vi "Sample Rate Trigger.vi"(8 "SampleDelay(in)":u32, 9 "Sample Rate (Hz)":dbl, 11 "Last Event mS":u32) -> (0 "Boolean":bool, 3 "Last Event mS":u32, 4 "Elapsed mS":u32, 6 "SampleDelay":u32)   [LabVIEW 2021]
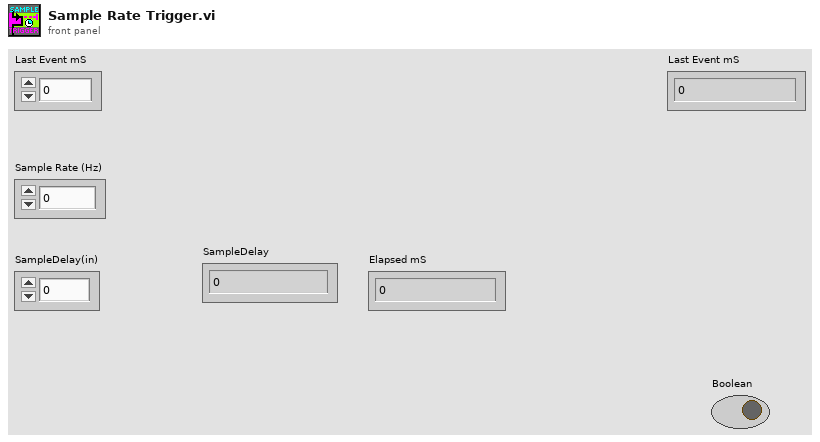
[diagram p1: front panel]
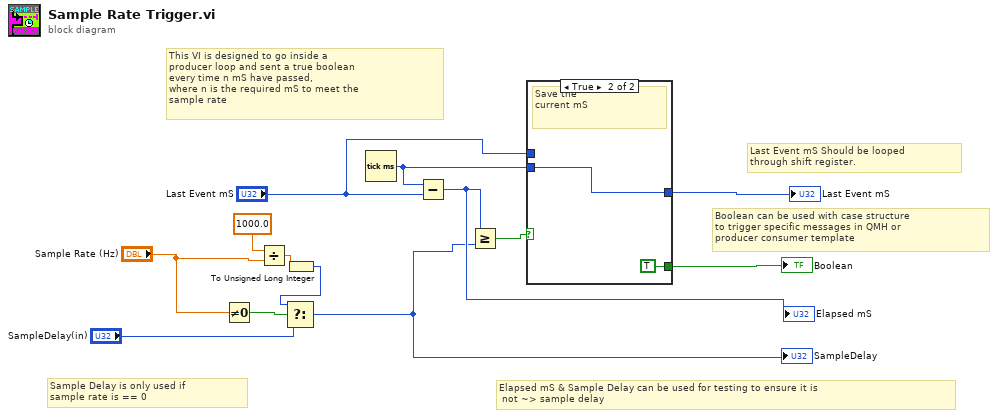
[diagram p0: block diagram]
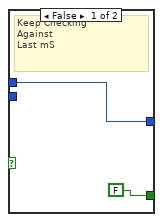
[diagram p2: hidden frame]
diagram:
  # "Sample Delay is only used if\nsample rate is == 0"
  # "Elapsed mS & Sample Delay can be used for testing to ensure it is\n not ~> sample delay"
  # "Boolean can be used with case structure\nto trigger specific messages in QMH or \nproducer consumer template"
  # "This VI is designed to go inside a\nproducer loop and sent a true boolean\nevery time n mS have passed, \nwhere n is the required mS to meet the \nsample rate"
  # "Last Event mS Should be looped\nthrough shift register."
  n1 = Not Equal To 0?(x="Sample Rate (Hz)") -> (x != 0?=w4:bool)
  n2 = Divide(x=1000.0, y="Sample Rate (Hz)") -> (x/y=w8:dbl)
  n3 = To Unsigned Long Integer(number=w8) -> (unsigned 32bit integer=w2:u32)
  n4 = Select(t=w2, s=w4, f="SampleDelay(in)") -> (s? t:f=w3:u32)
  "SampleDelay" <- w3
  n5 = Tick Count (ms)() -> (millisecond timer value=w11:u32)
  n6 = Subtract(x=w11, y="Last Event mS") -> (x-y=w6:u32)
  "Elapsed mS" <- w6
  n7 = Greater Or Equal?(x=w6, y=w3) -> (x >= y?=w9:bool)
  n8 = case shown="True" w9 {
    tunnel: [w15 w17] -> w10
    tunnel: w11 -> [_ w17]
    tunnel: "Last Event mS" -> [w15 _]
    tunnel: [FALSE TRUE] -> w13
    frame False {
      # "Keep Checking\nAgainst\nLast mS"
    }
    frame True {
      # "Save the \ncurrent mS"
    }
  }
  "Last Event mS" <- w10
  "Boolean" <- w13
